vi "Read Datalog file pathname.vi"() -> (0 "Datalog file pathname.":path, 1 "PASS/FAIL.":bool)   [LabVIEW 2010]
panel:
  # "No inputs:"
  # "Outputs."
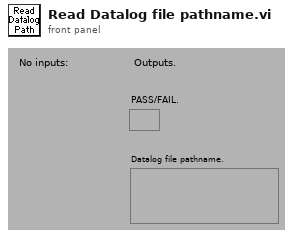
[diagram p1: front panel]
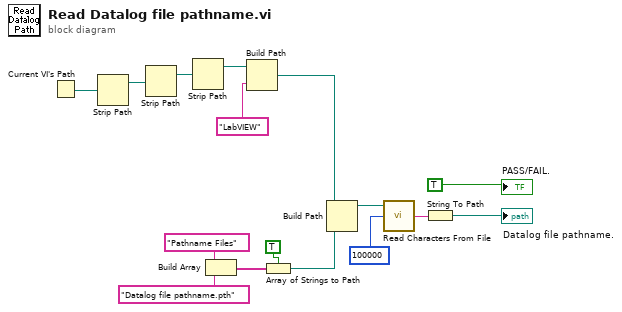
[diagram p0: block diagram]
diagram:
  n1 = Current VI's Path() -> (path=w6:path)
  n2 = Strip Path(path=w6) -> (stripped path=w5:path)  [unwired: 1 out]
  n3 = Strip Path(path=w5) -> (stripped path=w4:path)  [unwired: 1 out]
  n4 = Strip Path(path=w4) -> (stripped path=w3:path)  [unwired: 1 out]
  n5 = Build Array("Pathname Files", "Datalog file pathname.pth") -> (w16:string[])
  n6 = Build Path(base path=w3, name or relative path="LabVIEW") -> (appended path=w1:path)
  n7 = Array of Strings to Path(0:w16, 1:TRUE) -> (2:w9:path)
  n8 = Build Path(base path=w1, name or relative path=w9) -> (appended path=w10:path)
  n9 = call <vilib>:"Read Characters From File.vi"("file path (dialog if empty)"=w10, "number of characters (all:-1)"=100000) -> ("character string"=w12:string)  [unwired: 7 out]
  n10 = String To Path(string=w12) -> (path=→"Datalog file pathname.":path)
  "PASS/FAIL." <- TRUE
